vi "test BM Enable.vi"(8 "error in (no error)":errorcluster, 11 "BM Enable in":refnum<class "BM Enable.lvclass">) -> (0 "error out":errorcluster, 3 "BM Enable out":refnum<class "BM Enable.lvclass">)   [LabVIEW 2016, in "BM Enable.lvclass"]
uses:
  BM Enable.lvclass
  PPLs/FPGA Interface.lvlibp/FPGA Interface/FPGA Interface.lvclass
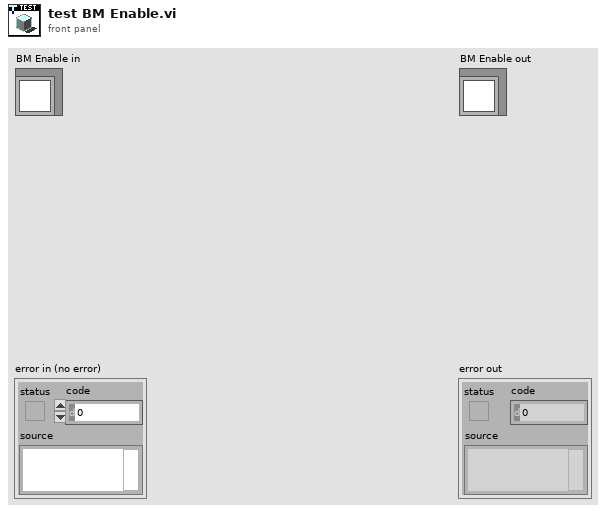
[diagram p1: front panel]
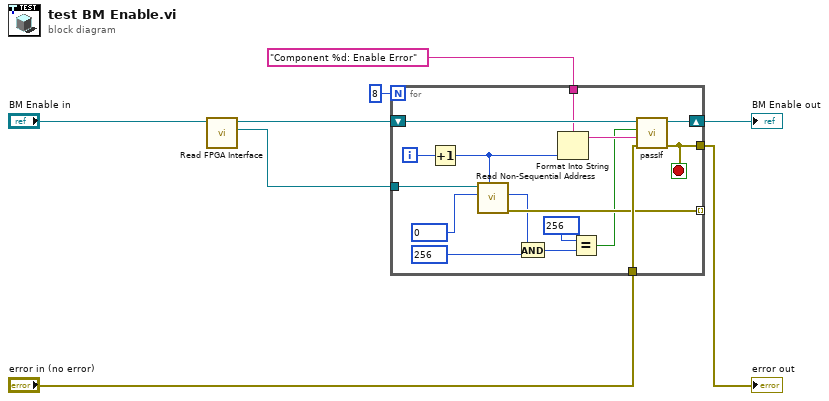
[diagram p0: block diagram]
diagram:
  n1 = call-dynamic "Read FPGA Interface.vi"("1553 Test in"="BM Enable in") -> ("FPGA Interface"=w3:refnum<class "FPGA Interface.lvclass">, "1553 Test out"=w4:refnum<class "BM Enable.lvclass">)  [unwired: 8 in, 1 out]
  n2 = for {
    N: 8 -> [_]
    tunnel: w3 -> [w24]
    shift-right: [w20] -> w6
    shift-left: w4 -> [w21]
    tunnel: "Component %d: Enable Error" ("custom report message (\"\")") -> [w19]
    tunnel: "error in (no error)" -> [w16]
    tunnel: [w15] -> w1
    tunnel: [w14] -> _ mode=indexing
    i -> [w23]
    stop <- w15 stop-if-true
    n3 = Increment(x=w23) -> (x+1=w18:i32)
    n4 = call-dynamic "Read Non-Sequential Address.vi"("Target IC (1-8)"=w18, "Address"=u16 0, "FPGA Interface in"=w24) -> ("error out"=w14:errorcluster, "Data"=w11:u16)  [unwired: 7 in]
    n5 = And(x=w11, y=u16 256) -> (x .and. y?=w12:u16)
    n6 = Format Into String(format string=w19, w18) -> (resulting string=w17:string)  [unwired: 2 in, 1 out]
    n7 = Equal?(x=u16 256, y=w12) -> (x = y?=w9:bool)
    n8 = call-dynamic "passIf.vi"("error in (no error)"=w16, "message (\"\")"=w17, "pass"=w9, "TestCase in"=w21) -> ("error out"=w15:errorcluster, "TestCase out"=w20:refnum<class "BM Enable.lvclass">)  [unwired: 6 in]
  }
  "error out" <- w1
  "BM Enable out" <- w6
